vi "Test Get When Filter Applied.vi"(8 "error in (no error)":errorcluster, 11 "Test Case In":refnum<class "Debugger Test.lvclass">) -> (0 "error out":errorcluster, 3 "Test Case Out":refnum<class "Debugger Test.lvclass">)   [LabVIEW 2020, in "Debugger Test.lvclass"]
uses:
  Debugger Test.lvclass
  C:/Program Files (x86)/National Instruments/LabVIEW 2020/vi.lib/Astemes/LUnit/Test Case.lvclass
  source/Debugger/Debugger.lvclass
  C:/Users/anton/Documents/GitHub/triarc-debugger/source/Process/Debug Process.lvclass
  source/Debug Data/Raw Debug Data.ctl
  source/Debug Data/Debug Data.lvclass/Debug Data.ctl
  source/Process/Debug Process.lvclass/Debug Process.ctl
  <vilib>/Astemes/LUnit/Test Case.lvclass/Test Case.ctl
  <vilib>/Astemes/LUnit/LUnit Assertion Result.lvclass/LUnit Assertion Result.ctl
  <vilib>/Astemes/LUnit/LUnit Test Case Result.lvclass/LUnit Test Case Result.ctl
  <vilib>/Astemes/LUnit/LUnit Method Result.lvclass/LUnit Method Result.ctl
  a5d622a0-a624-48a6-865c-c0c7a1259a45.vi
  <vilib>/AdvancedString/Delimited String to 1D String Array.vi
  source/Process/Public/Lifecycle/Get Lifecycle State.vi
  source/Process/Private/SubVIs/Wait for finish.vi
  source/Process/Protected/Messaging/Enqueue Message.vi
  source/Process/Private/SubVIs/Set Lifecycle State.vi
  <vilib>/Astemes/LUnit/Palette/Pass.vi
  <vilib>/Astemes/LUnit/Palette/Fail.vi
  <vilib>/Astemes/LUnit/Compare Variants.vi
  <vilib>/Astemes/LUnit/Describe Comparison.vi
  <vilib>/Astemes/LUnit/Set Assertion Type.vi
  <vilib>/Utility/error.llb/Clear Errors.vi
  <vilib>/Astemes/LUnit/Add test result.vi
  <vilib>/Astemes/LUnit/LUnit Write Passed.vi
  <vilib>/Astemes/LUnit/LUnit Write Message.vi
  <vilib>/Astemes/LUnit/LUnit Write Description.vi
  <vilib>/Astemes/LUnit/Variant to string.vi
  <vilib>/Astemes/LUnit/LUnit Write Assertion Type.vi
  <vilib>/Astemes/LUnit/LUnit Record Assertion Result.vi
  <vilib>/Astemes/LUnit/LUnit Aggregate Assertion Results.vi
  <vilib>/Astemes/LUnit/Assertion Result/LUnit Read Status.vi
  <vilib>/Astemes/LUnit/LUnit Read Message.vi
  <vilib>/Astemes/LUnit/LUnit Read Description.vi
  <vilib>/Astemes/LUnit/Method Result/LUnit Merge Status.vi
  <vilib>/Astemes/LUnit/LUnit Concatenate result strings.vi
  <vilib>/Utility/error.llb/Error Cluster From Error Code.vi
  <vilib>/Utility/Data Type/Get Type Information.vi
  <vilib>/Utility/LVClass/Get LV Class Name.vi
  source/Debug Data/Debug Data.lvclass
  <vilib>/Astemes/LUnit/LUnit Assertion Result.lvclass
  source/Process/Debug Process.lvclass
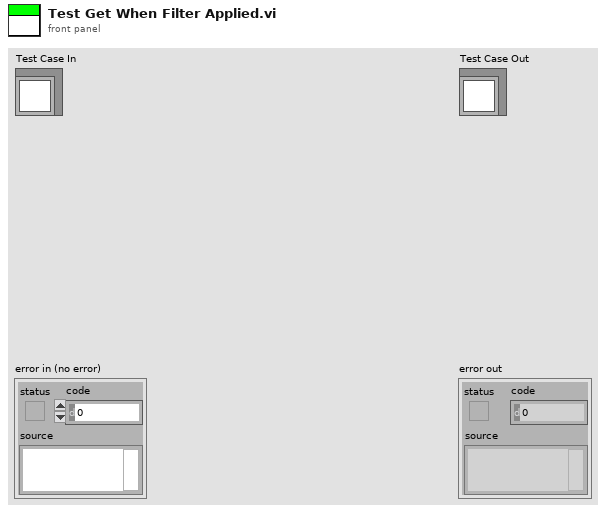
[diagram p1: front panel]
types:
  T1 = typedef "Debug Data.lvclass/Raw Debug Data.ctl" = cluster{"Action":string, "Call Chain":string, "Process":string, "Message":string, "Message Data":variant, "Time":dbl}
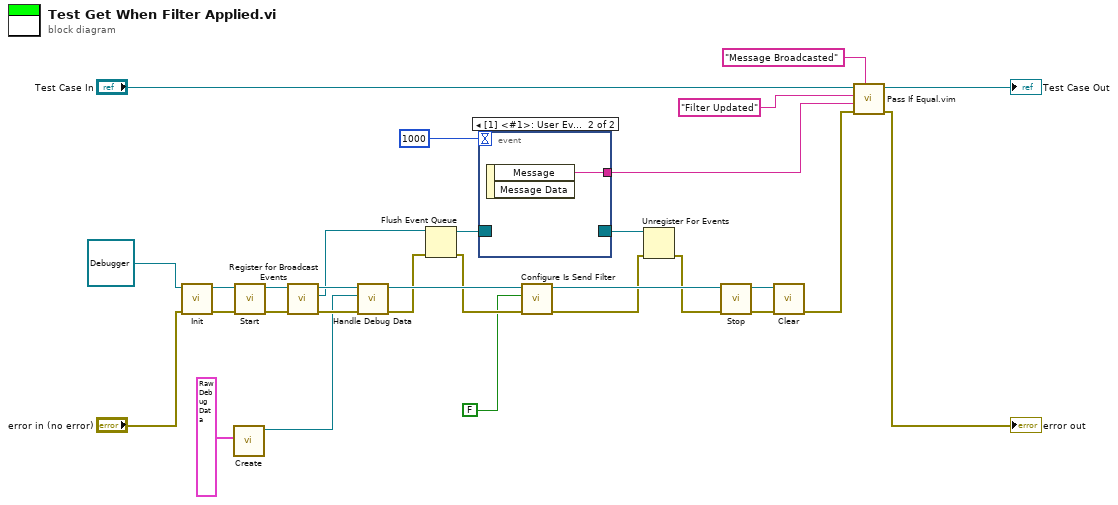
[diagram p0: block diagram]
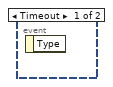
[diagram p2: hidden frame]
diagram:
  n1 = call-dynamic "Init.vi"("error in (no error)"="error in (no error)", "Process In"=refnum<class "Debugger.lvclass"> refnum ("Debug Data Event In 2")) -> ("error out"=w26:errorcluster, "Process Out"=w27:refnum<class "Debugger.lvclass">)  [unwired: 8 in]
  n2 = call "Create.vi"("Debug Data Cluster"=T1 {"Action"="", "Call Chain"="", "Process"="Test", "Message"="", "Message Data"=variant, "Time"=0.0}) -> ("Debug Data out"=w13:refnum<class "Debug Data.lvclass">)  [unwired: 9 in, 1 out]
  n3 = call "Start.vi"("error in (no error)"=w26, "Process In"=w27) -> ("error out"=w24:errorcluster, "Process Out"=w25:refnum<class "Debugger.lvclass">)  [unwired: 7 in, 1 out]
  n4 = call "Register for Broadcast Events.vi"("error in (no error)"=w24, "Process In"=w25) -> ("error out"=w23:errorcluster, "Event Registration Refnum Out"=w5:refnum<event-registration>, "Process Out"=w17:refnum<class "Debugger.lvclass">)  [unwired: 7 in]
  n5 = call-dynamic "Handle Debug Data.vi"("error in (no error)"=w23, "Debug Data.lvclass"=w13, "Debug Data Event In"=w17) -> ("error out"=w21:errorcluster, "Debug Data Event Out"=w22:refnum<class "Debugger.lvclass">)  [unwired: 7 in]
  n6 = Flush Event Queue(0:w5, 3:w21) -> (8:w4:refnum<event-registration>, 11:w6:errorcluster)  [unwired: 4 in, 1 out]
  n7 = event shown="[1] <#1>: User Event" {
    selector: w4 -> [_ _]
    dyn-events: [_ _] -> w10
    timeout: 1000 -> [_ _]
    tunnel: [_ w31] -> w9
    event Timeout {
      n8 = event-data() -> ()  [unwired: 1 in, 1 out]
    }
    event User Event {
      n9 = event-data() -> ("Message"=w31:string)  [unwired: 1 in, 1 out]
    }
  }
  n10 = call "Configure Is Send Filter.vi"("error in (no error)"=w6, "Show Send?"=FALSE, "Debugger In"=w22) -> ("error out"=w3:errorcluster, "Debugger Out"=w20:refnum<class "Debugger.lvclass">)  [unwired: 7 in]
  n11 = Unregister For Events(event registration refnum=w10, error in=w3) -> (error out=w2:errorcluster)
  n12 = call "Stop.vi"("error in (no error)"=w2, "Process In"=w20) -> ("error out"=w18:errorcluster, "Process Out"=w19:refnum<class "Debugger.lvclass">)  [unwired: 7 in, 1 out]
  n13 = call-dynamic "Clear.vi"("error in (no error)"=w18, "Process In"=w19) -> ("error out"=w14:errorcluster)  [unwired: 9 in]
  n14 = call "Pass If Equal.vim"("Description"="Message Broadcasted", "error in (no error)"=w14, "Actual"=w9, "Expected"="Filter Updated", "LUnit Test Case In"="Test Case In") -> ("error out"=→"error out":errorcluster, "LUnit Test Case Out"=→"Test Case Out":refnum<class "Debugger Test.lvclass">)  [unwired: 5 in]
